vi "Untitled 1.vi"() -> ()   [LabVIEW 2023]
uses:
  typedef_enum.ctl
panel:
  in  "STOP":bool
  out "STANJE":T1
  in  "10D":bool
  in  "5D":bool
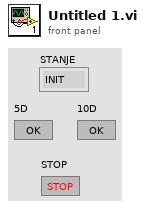
[diagram p1: front panel]
types:
  T1 = typedef "typedef_enum.ctl" = enum16{"INIT", "5D", "10D", "15D", "KUSUR", "20D"}
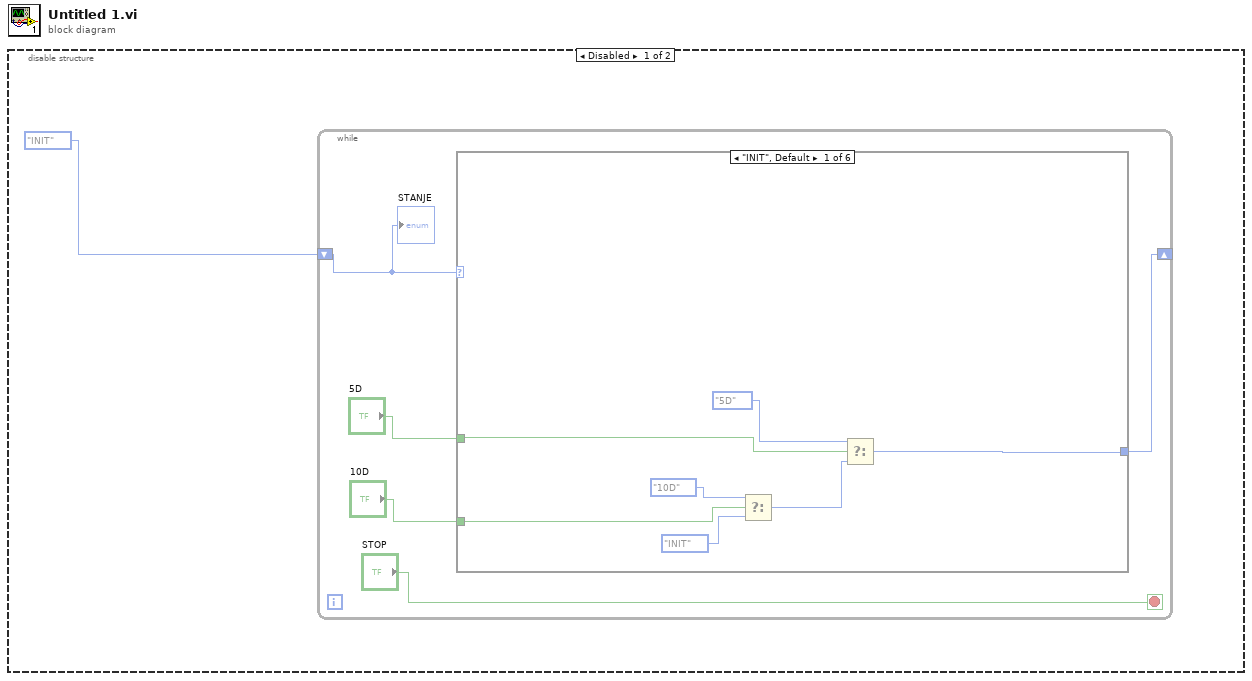
[diagram p0: block diagram]
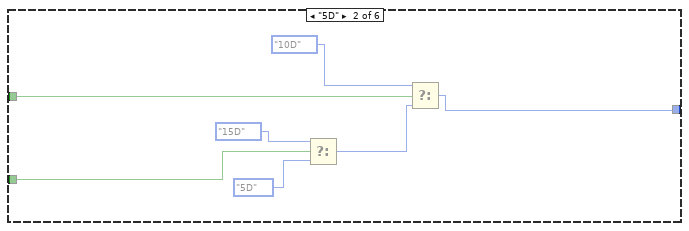
[diagram p2: hidden frame]
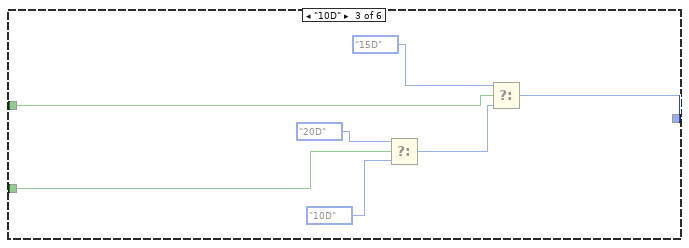
[diagram p3: hidden frame]
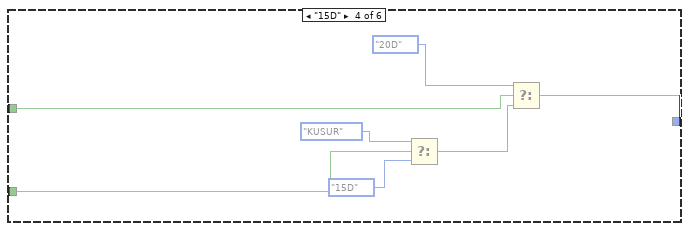
[diagram p4: hidden frame]
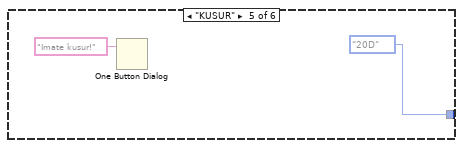
[diagram p5: hidden frame]
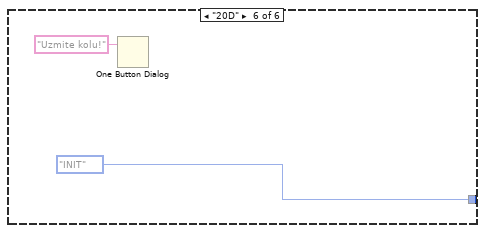
[diagram p6: hidden frame]
diagram:
  n1 = disable-structure shown="Disabled" {
    frame Disabled {
      n2 = while {
        shift-right: [w6] -> _
        shift-left: typedef_enum."INIT" ("Enum") -> [w5]
        stop <- "STOP" stop-if-true
        n3 = case shown="\"INIT\", Default" w5 {
          tunnel: "5D" -> [w9 w16 w23 w30 _ _]
          tunnel: "10D" -> [w8 w15 w22 w29 _ _]
          tunnel: [w7 w14 w21 w28 typedef_enum."20D" ("Enum") typedef_enum."INIT" ("Enum")] -> w6
          frame "INIT", Default {
            n4 = Select(t=typedef_enum."10D" ("Enum"), s=w8, f=typedef_enum."INIT") -> (s? t:f=w12:T1)
            n5 = Select(t=typedef_enum."5D" ("Enum"), s=w9, f=w12) -> (s? t:f=w7:T1)
          }
          frame "5D" {
            n6 = Select(t=typedef_enum."15D" ("Enum"), s=w15, f=typedef_enum."5D") -> (s? t:f=w19:T1)
            n7 = Select(t=typedef_enum."10D" ("Enum"), s=w16, f=w19) -> (s? t:f=w14:T1)
          }
          frame "10D" {
            n8 = Select(t=typedef_enum."20D" ("Enum"), s=w22, f=typedef_enum."10D") -> (s? t:f=w26:T1)
            n9 = Select(t=typedef_enum."15D" ("Enum"), s=w23, f=w26) -> (s? t:f=w21:T1)
          }
          frame "15D" {
            n10 = Select(t=typedef_enum."KUSUR" ("Enum"), s=w29, f=typedef_enum."15D") -> (s? t:f=w33:T1)
            n11 = Select(t=typedef_enum."20D" ("Enum"), s=w30, f=w33) -> (s? t:f=w28:T1)
          }
          frame "KUSUR" {
            n12 = One Button Dialog(message="Imate kusur!") -> ()  [unwired: 1 in, 1 out]
          }
          frame "20D" {
            n13 = One Button Dialog(message="Uzmite kolu!") -> ()  [unwired: 1 in, 1 out]
          }
        }
        "STANJE" <- w5
      }
    }
    frame Enabled {
    }
  }
